vi "IScanTemp.vi"(0 "PRIORLib.IScanIn":refnum<k7>) -> (1 "PRIORLib.IScanOut":refnum<k7>, 2 "error out":errorcluster, 3 "Return":i32, 4 "Temperature":sgl)   [LabVIEW 2011]
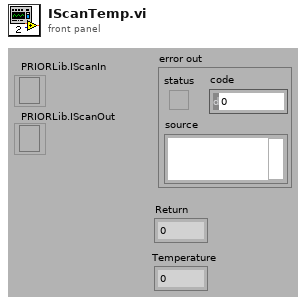
[diagram p1: front panel]
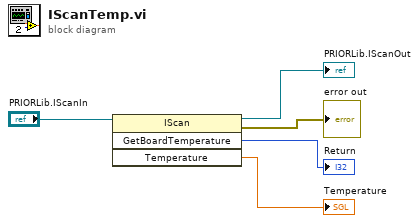
[diagram p0: block diagram]
diagram:
  n1 = invoke class="IScan" method="GetBoardTemperature"(reference="PRIORLib.IScanIn") -> (reference out=→"PRIORLib.IScanOut":refnum<k7>, error out=→"error out":errorcluster, "GetBoardTemperature"=→"Return":i32, "Temperature"=→"Temperature":sgl)  [unwired: 3 in]
